vi "Main FPGA 5-axis Servo 2.vi"() -> ()   [LabVIEW 2014]
uses:
  <vilib>/Motion/MotorControl/_s/nism.interpretControlRegister.stateTransition.ctl
  <vilib>/Motion/MotorControl/_s/nism.encoder.config.ctl
  <vilib>/Motion/MotorControl/_s/nism.encoder.incremental.config.ctl
  <vilib>/Motion/MotorControl/_s/nism.incremental.indexCriteria.ctl
  <vilib>/Motion/MotorControl/_s/nism.mdoMemoryOffsets.ctl
  <vilib>/Motion/MotorControl/_s/nism.pid.gains.fxp.18.ctl
  <vilib>/Motion/MotorControl/_s/nism.pi.v.outputRange.fxp.6.12.ctl
  <vilib>/Platform/TimedLoop/XDataNode/timing_clust.ctl
  <vilib>/Platform/TimedLoop/XDataNode/nitl_modes.ctl
  <vilib>/Platform/TimedLoop/XDataNode/wakeup.ctl
  <vilib>/Motion/MotorControl/_s/nism.digitalInputs.portA.ctl
  <vilib>/rvi/Emulation/niFpgaGetClockAttributes.vi
  <vilib>/rvi/Emulation/niFpgaSctlEmulationGetInTimedLoop.vi
  <vilib>/rvi/Emulation/niFpgaEmulationReportErrorSimple.vi
  Global FPGA.vi
  <vilib>/Motion/MotorControl/_s/nism.interpretControlRegister.indexed.vi
  <vilib>/rvi/Emulation/niFpgaProcessEmulError.vi
  <vilib>/Motion/MotorControl/_s/nism.mdo.read.encoder.vi
  <vilib>/Motion/MotorControl/_s/nism.mdo.read.positionLoopSyncData.vi
  <vilib>/Motion/MotorControl/_s/nism.mdo.read.splineData.vi
  <vilib>/Motion/MotorControl/_s/nism.mdo.read.single.vi
  <vilib>/Motion/MotorControl/_s/nism.generateStatusRegister.indexed.vi
  <vilib>/rvi/eio/common/nirviEmuTemplateMethod_errors.vi
  <vilib>/rvi/Emulation/niFpgaCriticalErrorInLSC.vi
  <vilib>/Motion/MotorControl/_s/nism.splineInterpolation.fxp.3.vi
  <vilib>/Motion/MotorControl/_s/nism.pid.simple.fxp.2.vi
  <vilib>/Motion/MotorControl/_s/nism.mdo.handler.indexed.vi
  <vilib>/Motion/MotorControl/_s/nism.digitalFilter.indexed.vi
  <vilib>/Motion/MotorControl/_s/nism.interpretDIOControl.portA.multiple.vi
  <vilib>/Motion/MotorControl/_s/nism.generateDIOStatus.portA.indexed.2.vi
  <vilib>/Motion/SoftMotion/Synchronization/nism.rioScan.generateSyncScan.vi
  <vilib>/Motion/MotorControl/_s/nism.incremental.p.2.vi
  <vilib>/eio/EIONode/EIONode.xnode
  <vilib>/rvi/Analysis/measure/butterworth/XNode/niFpgaButterworthFilter.xnode
  <vilib>/Platform/TimedLoop/XDataNode/XDataNode.xnode
  <vilib>/Motion/MotorControl/NI_SoftMotion_MotorControlIP.lvlib
  <vilib>/Platform/TimedLoop/XDataNode/XDNodeRunTimeDep.lvlib
  <vilib>/Motion/SoftMotion/Synchronization/NI_SoftMotion_Synchronization.lvlib
panel:
  in  "Reset Encoder":bool caption="reset"
  out "corrected period":u16
  out "AO Check":fxp<+/-,20,5>
  in  "AO Disabled":bool
  out "x-y":u32
  out "pos. error exceeded":bool
  out "position error":i16
  in  "AO 3":fxp<+/-,20,5>
  in  "AO 2":fxp<+/-,20,5>
  in  "AO 1":fxp<+/-,20,5>
  in  "AO 0":fxp<+/-,20,5>
  in  "AO Override?":bool
  in  "output range":T1={"output low"=-8.0, "output high"=8.0}
  in  "gains":T2
  in  "position error limit":i16=10000
  out "SE value":u32 caption="value"
  in  "Memory Type":T3=90 caption="mbox memory offsets" items=["1 / Current Loop Rate"=108, "Anti-Resonance Enable Velocity"=98, "Axis Control Mode"=88, "Axis Velocity Filter Coefficient 1"=60, "Axis Velocity Filter Coefficient 2"=61, "Axis Velocity Filter Coefficient 3"=62, "Axis Velocity Filter Frequency"=59, "Captured Index Position"=68, "Captured Position"=58, "Coefficient 0"=96, "Coefficient 1"=95, "Coefficient 2"=101, "Coefficient 3"=97, "Coefficient 4"=99, "Coefficient 5"=100, "Compare Mode"=81, "Compare Period"=32, "Compare Position"=55, "Config Sent"=82, "Control Register"=33, "Control Register State Transition"=57, "Current Loop I2T Constant"=38, "Current Loop I2T Current to Clamp to"=40, "Current Loop I2T Icont Limit Squared"=39, "Current Loop Integral Gain"=36, "Current Loop Proportional Gain"=35, "Current Loop Rate"=37, "Digital Input Digital Filter"=1, "Digital Output Safe State"=73, "Encoder Filter Rate (uS)"=92, "Encoder Index Active State"=65, "Encoder Index Reference Line A State"=66, "Encoder Index Reference Line B State"=67, "Encoder Line A Active State"=63, "Encoder Line B Active State"=64, "Encoder Velocity"=90, "Enforce Open-Loop Position Error Limit"=71, "Fault Codes"=45, "Fault Occurred"=41, "Forward Limit Digital Filter"=24, "Gain Set 2 Current Loop Integral Gain"=106, "Gain Set 2 Current Loop Proportional Gain"=107, "Home Switch Digital Filter"=26, "Maximum Position Error Exceeded"=69, "Motor Hall Angle 1"=12, "Motor Hall Angle 2"=13, "Motor Hall Angle 3"=14, "Motor Peak Current"=16, "Motor Peak Time"=17, "Motor Phase Current Offset(A)"=83, "Motor Phase Current Offset(B)"=84, "Motor Poles"=18, "Motor Rated Phase Current"=15, "Null"=0, "PWM Periods Per Tick"=94, "Position Capture Active State"=56, "Position Capture Condition"=30, "Position Capture Digital Filter"=31, "Position Compare Action"=27, "Position Compare Active State"=54, "Position Compare Pulse Width"=29, "Position Compare Safe State"=72, "Position Compare Window"=28, "Position Loop Period"=103, "Position Loop Position Error Limit"=70, "Position Loop Proportional Gain"=9, "Reverse Limit Digital Filter"=25, "Scan Period (nsec)"=104, "Spline Period/Trajectory Period"=44, "Spline Type"=42, "Status Register"=34, "Stepper Current Reduction Delay"=20, "Stepper Current Reduction Percentage"=19, "Stepper Microstepping Rate"=21, "Stepper Minimum Pulse Width"=22, "Stepper Reduced Current"=85, "Stepper Spline Loop Period"=23, "Torque Smoothing Gain"=102, "Torque Smoothing Phase"=105, "Trajectory Period/Spline Period"=43]
  in  "Encoder filter value (us) Manual":u16=2000
  out "encoder config":T4
  in  "Velocity Filter Active?":bool
  in  "Encoder Config (Manual)":T4={"active states"={"line a active high?"=FALSE, "line b active high?"=FALSE, "index active high?"=FALSE}, "index criteria"={"a"=FALSE, "b"=FALSE, "z"=FALSE}, "vel. filter coeffs."=[0, 0, 0]} caption="encoder config"
  out "Home Limits":bool[](array[boolean])
  out "Fwd Limits":bool[](array[boolean])
  out "Rev Limits":bool[](array[boolean])
  out "Drive Enable":bool[](array[boolean])
  in  "Enable Watchdog":bool
  in  "Pet Watchdog":bool
  in  "Watchdog Timeout Period (ticks)":u64=40000000 format="%.0p"
  out "Watchdog Timed Out?":bool
  out "Time Since Last Pet":u64
  in  "Enable value":bool
  in  "Drive Enable override?":bool
  out "State":T7=enum."Start --> Initializing" caption="state transition"
  in  "Sync Value":bool
  in  "Sync Enable override?":bool
  in  "Invert direction?":bool
  out "Sync is Fault":bool
  out "Sync is Locked":bool
  # "Synchronization Loop"
  # "Control Status Loop"
  # "Notes: \n1. This VI provides the communication interface between the NI SoftMotion Engine and the LabVIEW FPGA Module. You must compile this VI for a specific FPGA target before use. After compiling, run the VI before running any of the Express VI examples. For information on moving this example to another FPGA target, refer to ni.com/info and enter info code fpgaex.\n\n2. Only use the Reset Axis button if you are unable to communicate with the axis by any other means. This button resets the device state machine and other VIs to a known state. After resetting the axis, switch the NI Scan Engine from Active Mode to Configuration Mode, then back to Active Mode, before attempting to enable the axis."
  # "(These two buttons \nare for testing\npurposes.)"
  # "(These two buttons \nare for testing\npurposes.)"
  # "Step/Direction Loop"
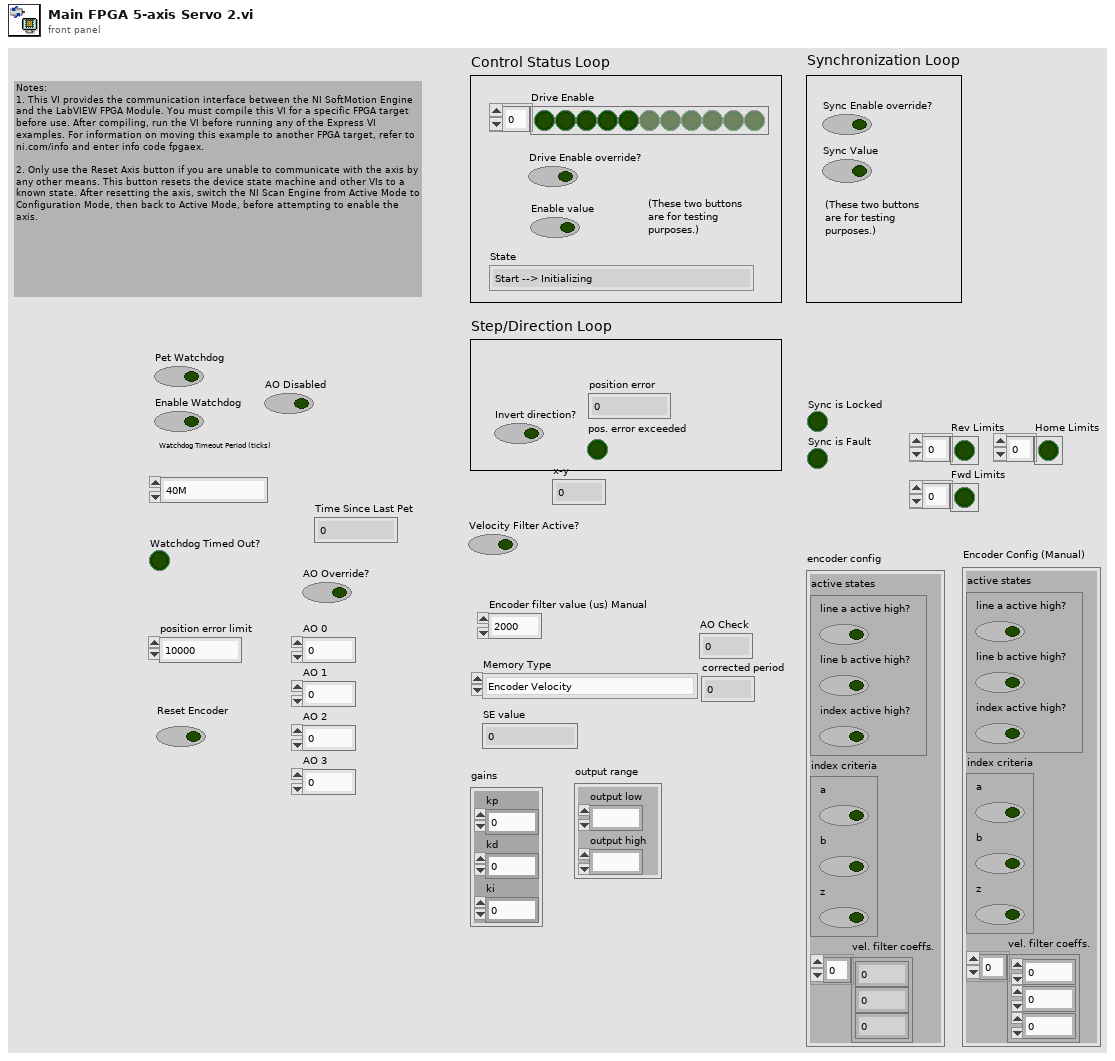
[diagram p1: front panel]
types:
  T1 = typedef "NI_SoftMotion_MotorControlIP.lvlib/nism.pi.v.outputRange.fxp.6.12.ctl" = cluster{"output low":fxp<+/-,18,6>, "output high":fxp<+/-,18,6>}
  T2 = typedef "NI_SoftMotion_MotorControlIP.lvlib/nism.pid.gains.fxp.18.ctl" = cluster{"kp":fxp<+,18,7>, "kd":fxp<+,18,7>, "ki":fxp<+,18,0>}
  T3 = typedef "NI_SoftMotion_MotorControlIP.lvlib/nism.mdoMemoryOffsets.ctl" = u16
  T4 = typedef "NI_SoftMotion_MotorControlIP.lvlib/nism.encoder.config.ctl" = cluster{"active states":T5, "index criteria":T6, "vel. filter coeffs.":i32[]}
  T5 = typedef "NI_SoftMotion_MotorControlIP.lvlib/nism.encoder.incremental.config.ctl" = cluster{"line a active high?":bool, "line b active high?":bool, "index active high?":bool}
  T6 = typedef "NI_SoftMotion_MotorControlIP.lvlib/nism.incremental.indexCriteria.ctl" = cluster{"a":bool, "b":bool, "z":bool}
  T7 = typedef "NI_SoftMotion_MotorControlIP.lvlib/nism.interpretControlRegister.stateTransition.ctl" = enum8{"Invalid", "Start --> Initializing", "Initializing --> Disabled", "Disabled --> Ready To Switch On", "Ready To Switch On --> Switched On", "Ready To Switch On --> Disable", "Switched On --> Operation Enable", "Switched On --> Ready To Switch On", "Switched On --> Disabled", "Operation Enable --> Switched On", "Operation Enable --> Ready To Switch On", "Operation Enable --> Disabled", "Fault --> Disabled", "Any --> Fault", "None"}
  T8 = typedef "NI_SoftMotion_Synchronization.lvlib/nism.softmotionScan.timerConfig.ctl" = cluster{"target period (clocks)":u16, "host period / target period":u16}
  T9 = typedef "NI_SoftMotion_Synchronization.lvlib/nism.softmotionScan.timerControl.ctl" = cluster{"sm scan":bool, "sm scan count":u32, "sm scan enabled":bool}
  T10 = typedef "NI_SoftMotion_MotorControlIP.lvlib/nism.mdo.splineData.ctl" = cluster{"spline type":T11, "traj per/spline per":u16, "spline per/traj per":fxp<+,32,0>}
  T11 = typedef "NI_SoftMotion_MotorControlIP.lvlib/nism.splineInterpolation.type.ctl" = u16
  T12 = typedef "NI_SoftMotion_MotorControlIP.lvlib/nism.digitalInputs.portA.ctl" = cluster{"reverse limit":bool, "forward limit":bool, "home switch":bool, "digital input 0":bool, "digital input 1":bool, "digital input 2":bool, "digital input 3":bool}
  T13 = typedef "NI_SoftMotion_MotorControlIP.lvlib/nism.dio.portA.config.2.ctl" = cluster{"digital filter (us)":u16[], "safe state":T14[]}
  T14 = typedef "nism.safeStates.ctl" = enum8{"Low", "High", "No Change"}
  T15 = typedef "XDNodeRunTimeDep.lvlib/timing_clust.ctl" = cluster{"Expected End [f-1]":u64, "Actual End [f-1]":u64, "Finished Late? [f-1]":bool, "Expected End [i-1]":u64, "Actual End [i-1]":u64, "Finished Late? [i-1]":bool, "Expected Start [i]":u64, "Actual Start [i]":u64, "Expected Start [f]":u64, "Actual Start [f]":u64, "Source Name":string, "Structure Name":string, "Period":i64, "Deadline":i64, "Offset":i64, "Start":i64, "Priority":i32, "Timeout":i32, "Mode":T16, "Wakeup Reason":T17, "Error":errorcluster, "Source Type":string, "Secondary Source Type":string, "Global End Time":u64, "Global Start Time":u64, "Frame Duration":u64, "Iteration Duration":u64, "Assigned CPU":i32, "I/O Scan Engine Mode":u32}
  T16 = typedef "XDNodeRunTimeDep.lvlib/nitl_modes.ctl" = enum32{"No Change", "Process missed periods, maintain original phase", "Discard missed periods, maintain original phase", "Process missed periods, ignore original phase", "Discard missed periods, ignore original phase"}
  T17 = typedef "XDNodeRunTimeDep.lvlib/wakeup.ctl" = enum32{"Normal", "Aborted", "Asynchronous wakeup", "Timing source error", "Timed loop error", "Timeout"}
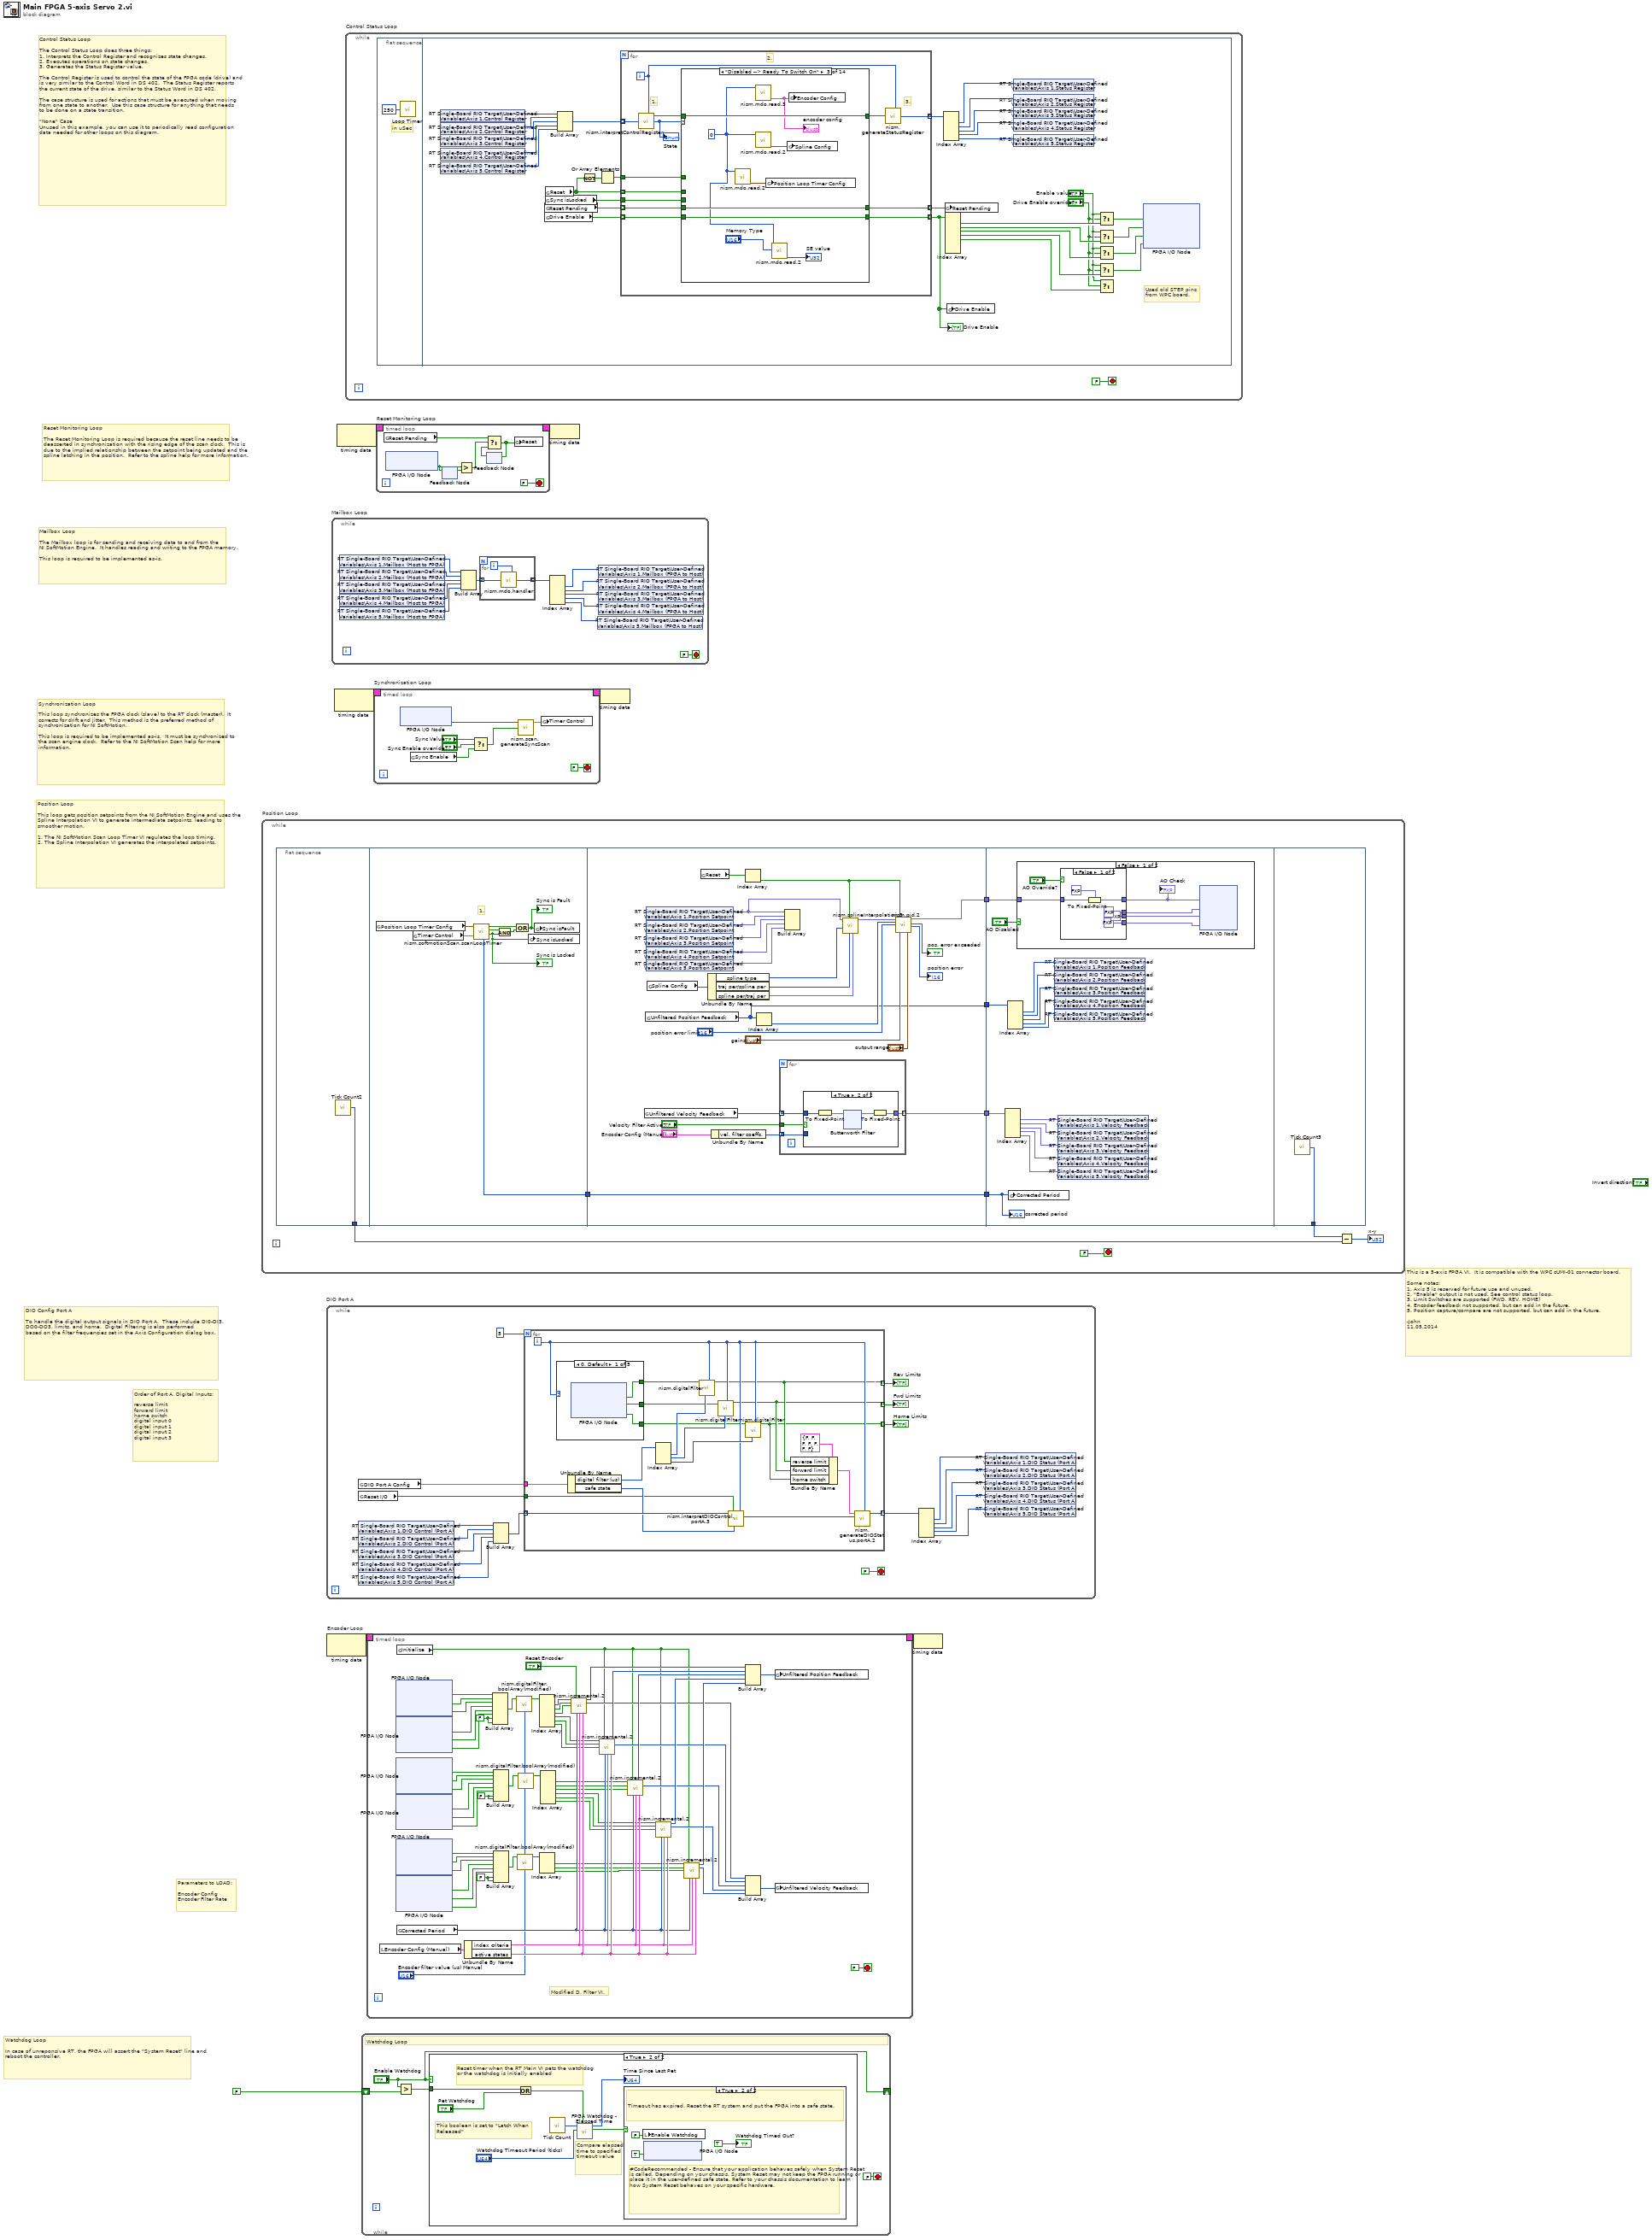
[diagram p0: block diagram]
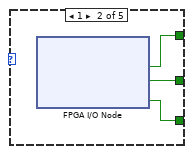
[diagram p2: hidden frame]
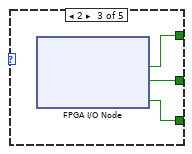
[diagram p3: hidden frame]
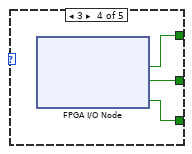
[diagram p4: hidden frame]
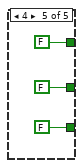
[diagram p5: hidden frame]
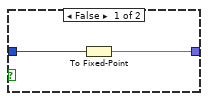
[diagram p8: hidden frame]
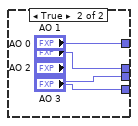
[diagram p9: hidden frame]
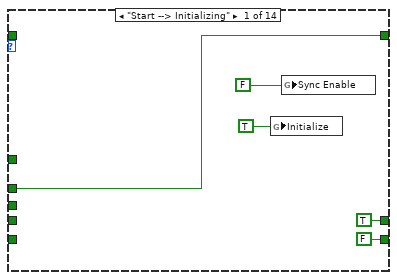
[diagram p11: hidden frame]
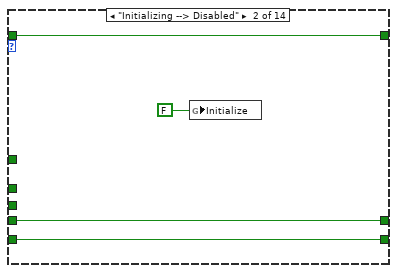
[diagram p12: hidden frame]
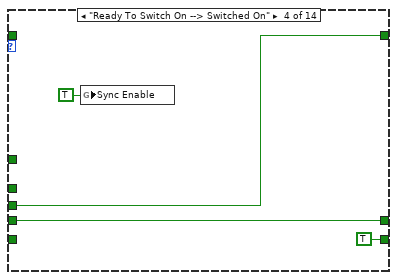
[diagram p13: hidden frame]
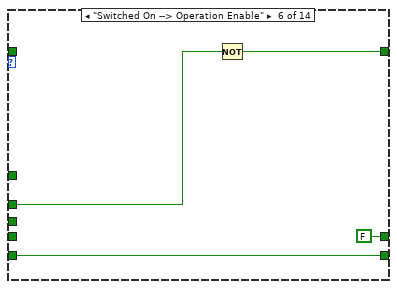
[diagram p15: hidden frame]
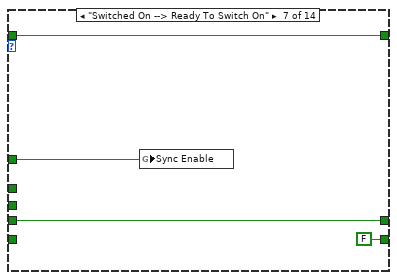
[diagram p16: hidden frame]
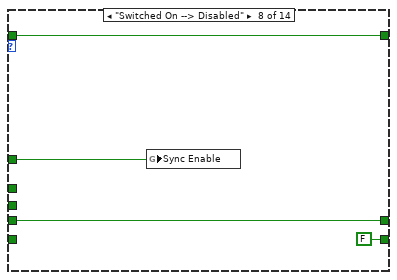
[diagram p17: hidden frame]
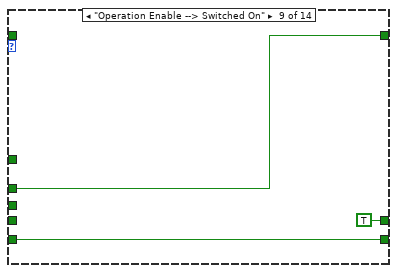
[diagram p18: hidden frame]
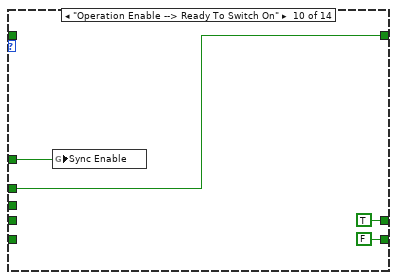
[diagram p19: hidden frame]
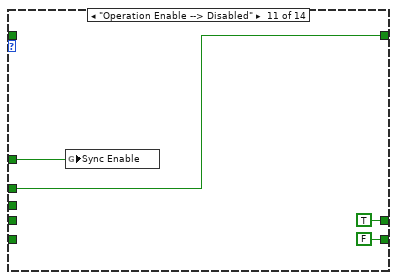
[diagram p20: hidden frame]
diagram:
  # "Parameters to LOAD:\n\nEncoder Config\nEncoder Filter Rate"
  # "This is a 5-axis FPGA VI.  It is compatible with the WPC cUMI-01 connector board.\n\nSome notes:\n1. Axis 5 is reserved for future use and unused.\n2. \"Enable\" output is not used. See control status loop.\n3. Limit Switches are supported (FWD, REV, HOME)\n4. Encoder feedback not supported, but can add in the future.\n5. Position capture/compare are not supported, but can add in the future.\n\n-John\n11.05.2014"
  # "DIO Config Port A\n\nTo handle the digital output signals in DIO Port A.  These include DI0-DI3, DO0-DO3, limits, and home.  Digital Filtering is also performed\nbased on the filter frequencies set in the Axis Configuration dialog box."
  # "Order of Port A, Digital Inputs:\n\nreverse limit\nforward limit\nhome switch\ndigital input 0\ndigital input 1\ndigital input 2\ndigital input 3"
  # "Watchdog Loop\n\nIn case of unreponsive RT, the FPGA will assert the \"System Reset\" line and reboot the controller."
  # "Position Loop\n\nThis loop gets position setpoints from the NI SoftMotion Engine and uses the Spline Interpolation VI to generate intermediate setpoints, leading to smoother motion.\n\n1. The NI SoftMotion Scan Loop Timer VI regulates the loop timing. \n2. The Spline Interpolation VI generates the interpolated setpoints."
  # "Synchronization Loop\n\nThis loop synchronizes the FPGA clock (slave) to the RT clock (master).  It corrects for drift and jitter.  This method is the preferred method of synchronization for NI SoftMotion.\n\nThis loop is required to be implemented as-is.  It must be synchronized to the scan engine clock.  Refer to the NI SoftMotion Scan help for more information."
  # "Mailbox Loop\n\nThe Mailbox loop is for sending and receiving data to and from the \nNI SoftMotion Engine.  It handles reading and writing to the FPGA memory.\n\nThis loop is required to be implemented as-is."
  # "Reset Monitoring Loop\n\nThe Reset Monitoring Loop is required because the reset line needs to be deasserted in synchronization with the rising edge of the scan clock.  This is due to the implied relationship between the setpoint being updated and the spline latching in the position.  Refer to the spline help for more information."
  # "Control Status Loop\n\nThe Control Status Loop does three things:\n1. Interprets the Control Register and recognizes state changes.\n2. Executes operations on state changes.\n3. Generates the Status Register value.\n\nThe Control Register is used to control the state of the FPGA code (drive) and is very similar to the Control Word in DS 402.  The Status Register reports the current state of the drive, similar to the Status Word in DS 402.\n\nThe case structure is used for actions that must be executed when moving from one state to another.  Use this case structure for anything that needs to be done on a state transition.\n\n\"None\" Case\nUnused in this example, you can use it to periodically read configuration data needed for other loops on this diagram."
  n1 = while "Position Loop" {
    stop <- FALSE stop-if-true
    n2 = flat-sequence {
      tunnel: [w17] -> w10
      tunnel: [w18] -> w14
      tunnel: [w46] -> w15
      tunnel: w14 -> [w46]
      tunnel: [w27] -> w13
      tunnel: [w39] -> w12
      tunnel: [w26] -> w8
      tunnel: w15 -> [w85]
      tunnel: w13 -> [w84]
      tunnel: w12 -> [w78]
      tunnel: w8 -> [w72]
      tunnel: [w102] -> w11
      frame #0 {
        n3 = call "Tick Count2"() -> ("Tick Count(Ticks)"=w17:u32)
      }
      frame #1 {
        # "1."
        n4 = global read "Global FPGA.vi" "Position Loop Timer Config"() -> (w20:T8)
        n5 = global read "Global FPGA.vi" "Timer Control"() -> (w19:T9)
        n6 = call <vilib>:"nism.softmotionScan.scanLoopTimer.vi"("timer control"=w19, "timer config"=w20) -> ("scan running?"=w22:bool, "finished late?"=w24:bool, "fault occurred?"=w25:bool, "corrected period"=w18:u16)  [unwired: 5 in, 1 out]
        "Sync is Locked" <- w22
        n7 = Compound Arithmetic op=AND(w24, w22) -> (w23:bool)
        n8 = Compound Arithmetic op=OR(w25, w23) -> (w21:bool)
        "Sync is Fault" <- w21
        n9 = global write "Global FPGA.vi" "Sync isLocked"(w22) -> ()
        n10 = global write "Global FPGA.vi" "Sync isFault"(w21) -> ()
      }
      frame #2 {
        n11 = global read "Global FPGA.vi" "Unfiltered Velocity Feedback"() -> (w40:i16[])
        n12 = global read "Global FPGA.vi" "Unfiltered Position Feedback"() -> (w27:i32[])
        n13 = shared-variable "RT Single-Board RIO Target\\User-Defined Variables\\Axis 1.Position Setpoint"() -> (w30:fxp<+/-,64,32>)  [unwired: 1 in, 1 out]
        n14 = shared-variable "RT Single-Board RIO Target\\User-Defined Variables\\Axis 2.Position Setpoint"() -> (w45:fxp<+/-,64,32>)  [unwired: 1 in, 1 out]
        n15 = shared-variable "RT Single-Board RIO Target\\User-Defined Variables\\Axis 3.Position Setpoint"() -> (w44:fxp<+/-,64,32>)  [unwired: 1 in, 1 out]
        n16 = shared-variable "RT Single-Board RIO Target\\User-Defined Variables\\Axis 4.Position Setpoint"() -> (w43:fxp<+/-,64,32>)  [unwired: 1 in, 1 out]
        n17 = shared-variable "RT Single-Board RIO Target\\User-Defined Variables\\Axis 5.Position Setpoint"() -> (w42:fxp<+/-,64,32>)  [unwired: 1 in, 1 out]
        n18 = global read "Global FPGA.vi" "Spline Config"() -> (w48:T10)
        n19 = global read "Global FPGA.vi" "Reset"() -> (w32:bool[])
        n20 = Unbundle By Name(w48) -> ("spline type"=w51:T11, "traj per/spline per"=w50:u16, "spline per/traj per"=w49:fxp<+,32,0>)
        n21 = Unbundle By Name("Encoder Config (Manual)") -> ("vel. filter coeffs."=w41:i32[])
        n22 = Index Array(array=w32) -> (element=w31:bool)  [unwired: 1 in]
        n23 = Index Array(array=w27) -> (element=w33:i32)  [unwired: 1 in]
        n24 = for {
          tunnel: "Velocity Filter Active?" -> [w55]
          tunnel: w41 -> [w54] mode=indexing
          tunnel: w40 -> [w53] mode=indexing
          tunnel: [w52] -> w39 mode=indexing
          n25 = case shown="True" w55 {
            tunnel: w53 -> [w57 w61]
            tunnel: w54 -> [_ _]
            tunnel: [w56 w59] -> w52
            frame False {
              n26 = To Fixed-Point(number=w57) -> (fixed-point=w56:fxp<+/-,64,32>)  [unwired: 1 in]
            }
            frame True {
              n27 = To Fixed-Point(number=w61) -> (fixed-point=w60:fxp<+/-,16,16>)  [unwired: 1 in]
              n28 = xnode "Butterworth Filter"("input data"=w60) -> ("output data"=w58:fxp<+/-,16,16>)  [unwired: 2 in, 1 out]
              n29 = To Fixed-Point(number=w58) -> (fixed-point=w59:fxp<+/-,64,32>)  [unwired: 1 in]
            }
          }
        }
        n30 = Build Array(w30, w45, w44, w43, w42) -> ()  [unwired: 1 out]
        n31 = call-poly <vilib>:"nism.splineInterpolation.3.vi"("1 / calls per sample"=w49, "calls per sample"=w50, "reset"=w31, "spline type"=w51, "x"=w30) -> ("xi"=w47:fxp<+/-,64,32>)  [unwired: 5 in, 1 out]
        n32 = call-poly <vilib>:"nism.pid.2.vi"("position setpoint"=w47, "position feedback"=w33, "position error limit"="position error limit", "reset"=w31, "gains"="gains", "output range"="output range") -> ("current setpoint"=w26:fxp<+/-,18,6>, "pos. error exceeded"=→"pos. error exceeded":bool, "position error"=→"position error":i16)  [unwired: 11 in]
      }
      frame #3 {
        n33 = Index Array(array=w78) -> (element #1=w77:fxp<+/-,64,32>, element #2=w76:fxp<+/-,64,32>, element #3=w75:fxp<+/-,64,32>, element #4=w74:fxp<+/-,64,32>, element #5=w73:fxp<+/-,64,32>)  [unwired: 5 in]
        n34 = Index Array(array=w84) -> (element #1=w83:i32, element #2=w82:i32, element #3=w81:i32, element #4=w80:i32, element #5=w79:i32)  [unwired: 5 in]
        n35 = global write "Global FPGA.vi" "Corrected Period"(w85) -> ()
        n36 = case shown="False" "AO Disabled" {
          tunnel: w72 -> [w86 _]
          frame False {
            n37 = case shown="False" "AO Override?" {
              tunnel: [w93 "AO 0"] -> w90
              tunnel: [fxp<+/-,20,5> 0.0 ("AO 1") "AO 1"] -> w89
              tunnel: [fxp<+/-,20,5> 0.0 ("AO 2") "AO 2"] -> w88
              tunnel: [fxp<+/-,20,5> 0.0 ("AO 3") "AO 3"] -> w87
              tunnel: w86 -> [w92 _]
              frame False {
                n38 = To Fixed-Point(fixed-point type=fxp<+/-,20,5> 0.0 ("AO 1"), number=w92) -> (fixed-point=w93:fxp<+/-,20,5>)
              }
              frame True {
              }
            }
            "AO Check" <- w90
            n39 = xnode "FPGA I/O Node"("AO0"=w90, "AO1"=w89, "AO2"=w88, "AO3"=w87) -> ()  [unwired: 4 in, 4 out]
          }
          frame True {
          }
        }
        n40 = shared-variable "RT Single-Board RIO Target\\User-Defined Variables\\Axis 1.Position Feedback"(w83) -> ()  [unwired: 1 in, 1 out]
        n41 = shared-variable "RT Single-Board RIO Target\\User-Defined Variables\\Axis 2.Position Feedback"(w82) -> ()  [unwired: 1 in, 1 out]
        n42 = shared-variable "RT Single-Board RIO Target\\User-Defined Variables\\Axis 3.Position Feedback"(w81) -> ()  [unwired: 1 in, 1 out]
        n43 = shared-variable "RT Single-Board RIO Target\\User-Defined Variables\\Axis 4.Position Feedback"(w80) -> ()  [unwired: 1 in, 1 out]
        n44 = shared-variable "RT Single-Board RIO Target\\User-Defined Variables\\Axis 5.Position Feedback"(w79) -> ()  [unwired: 1 in, 1 out]
        n45 = shared-variable "RT Single-Board RIO Target\\User-Defined Variables\\Axis 1.Velocity Feedback"(w77) -> ()  [unwired: 1 in, 1 out]
        n46 = shared-variable "RT Single-Board RIO Target\\User-Defined Variables\\Axis 2.Velocity Feedback"(w76) -> ()  [unwired: 1 in, 1 out]
        n47 = shared-variable "RT Single-Board RIO Target\\User-Defined Variables\\Axis 3.Velocity Feedback"(w75) -> ()  [unwired: 1 in, 1 out]
        n48 = shared-variable "RT Single-Board RIO Target\\User-Defined Variables\\Axis 4.Velocity Feedback"(w74) -> ()  [unwired: 1 in, 1 out]
        n49 = shared-variable "RT Single-Board RIO Target\\User-Defined Variables\\Axis 5.Velocity Feedback"(w73) -> ()  [unwired: 1 in, 1 out]
        "corrected period" <- w85
      }
      frame #4 {
        n50 = call "Tick Count3"() -> ("Tick Count(Ticks)"=w102:u32)
      }
    }
    n51 = Subtract(x=w11, y=w10) -> (x-y=→"x-y":u32)
  }
  n52 = while "DIO Port A" {
    stop <- FALSE stop-if-true
    n53 = global read "Global FPGA.vi" "DIO Port A Config"() -> (w120:T13)
    n54 = global read "Global FPGA.vi" "Reset I/O"() -> (w119:bool)
    n55 = shared-variable "RT Single-Board RIO Target\\User-Defined Variables\\Axis 1.DIO Control (Port A)"() -> (w117:u32)  [unwired: 1 in, 1 out]
    n56 = shared-variable "RT Single-Board RIO Target\\User-Defined Variables\\Axis 2.DIO Control (Port A)"() -> (w116:u32)  [unwired: 1 in, 1 out]
    n57 = shared-variable "RT Single-Board RIO Target\\User-Defined Variables\\Axis 3.DIO Control (Port A)"() -> (w115:u32)  [unwired: 1 in, 1 out]
    n58 = shared-variable "RT Single-Board RIO Target\\User-Defined Variables\\Axis 4.DIO Control (Port A)"() -> (w114:u32)  [unwired: 1 in, 1 out]
    n59 = shared-variable "RT Single-Board RIO Target\\User-Defined Variables\\Axis 5.DIO Control (Port A)"() -> (w113:u32)  [unwired: 1 in, 1 out]
    n60 = Build Array(w117, w116, w115, w114, w113) -> (w112:u32[])
    n61 = for {
      N: 5 -> [_]
      tunnel: [w139] -> w106 mode=indexing
      tunnel: w112 -> [w138] mode=indexing
      tunnel: w120 -> [w135]
      tunnel: w119 -> [w133]
      tunnel: [w124] -> w105 mode=indexing
      tunnel: [w123] -> w104 mode=indexing
      tunnel: [w122] -> w103 mode=indexing
      i -> [w128]
      n62 = case shown="0, Default" w128 {
        tunnel: [w143 w146 w149 w152 FALSE ("RMC/DIO44")] -> w127
        tunnel: [w141 w144 w147 w150 FALSE ("RMC/DIO61")] -> w126
        tunnel: [w142 w145 w148 w151 FALSE ("RMC/DIO77")] -> w125
        frame 0, Default {
          n63 = xnode "FPGA I/O Node"() -> ("RMC/DIO29"=w143:bool, "RMC/DIO93"=w142:bool, "RMC/DIO11"=w141:bool)  [unwired: 3 in, 3 out]
        }
        frame 1 {
          n64 = xnode "FPGA I/O Node"() -> ("RMC/DIO44"=w146:bool, "RMC/DIO77"=w145:bool, "RMC/DIO61"=w144:bool)  [unwired: 3 in, 3 out]
        }
        frame 2 {
          n65 = xnode "FPGA I/O Node"() -> ("RMC/DIO31"=w149:bool, "RMC/DIO95"=w148:bool, "RMC/DIO13"=w147:bool)  [unwired: 3 in, 3 out]
        }
        frame 3 {
          n66 = xnode "FPGA I/O Node"() -> ("RMC/DIO47"=w152:bool, "RMC/DIO46"=w151:bool, "RMC/DIO79"=w150:bool)  [unwired: 3 in, 3 out]
        }
        frame 4 {
        }
      }
      n67 = Unbundle By Name(w135) -> ("digital filter (us)"=w129:u16[], "safe state"=w134:T14[])
      n68 = Index Array(array=w129) -> (element #1=w130:u16, element #2=w131:u16, element #3=w132:u16)  [unwired: 3 in]
      n69 = call-poly <vilib>:"nism.digitalFilter.vi"("index"=w128, "filter value (us)"=w130, "input signal"=w127) -> ("output signal"=w124:bool)  [unwired: 8 in]
      n70 = call-poly <vilib>:"nism.digitalFilter.vi"("index"=w128, "filter value (us)"=w131, "input signal"=w125) -> ("output signal"=w123:bool)  [unwired: 8 in]
      n71 = call-poly <vilib>:"nism.interpretDIOControl.portA.3.vi"("index"=w128, "safe state"=w134, "reset"=w133, "dio control(port a)"=w138) -> ("reset latches"=w140:u8)  [unwired: 6 in, 1 out]
      n72 = call-poly <vilib>:"nism.digitalFilter.vi"("index"=w128, "filter value (us)"=w132, "input signal"=w126) -> ("output signal"=w122:bool)  [unwired: 8 in]
      n73 = Bundle By Name(cluster=T12 {"reverse limit"=FALSE, "forward limit"=FALSE, "home switch"=FALSE, "digital input 0"=FALSE, "digital input 1"=FALSE, "digital input 2"=FALSE, "digital input 3"=FALSE} ("$(driveInterface.digitalInputs.shortName)"), "reverse limit"=w124, "forward limit"=w123, "home switch"=w122) -> (w136:T12)
      n74 = call-poly <vilib>:"nism.generateDIOStatus.portA.2.vi"("index"=w128, "reset latches"=w140, "digital inputs"=w136) -> ("dio status(port a)"=w139:u32)  [unwired: 8 in]
    }
    "Rev Limits" <- w105
    "Fwd Limits" <- w104
    "Home Limits" <- w103
    n75 = Index Array(array=w106) -> (element #1=w111:u32, element #2=w110:u32, element #3=w109:u32, element #4=w108:u32, element #5=w107:u32)  [unwired: 5 in]
    n76 = shared-variable "RT Single-Board RIO Target\\User-Defined Variables\\Axis 1.DIO Status (Port A)"(w111) -> ()  [unwired: 1 in, 1 out]
    n77 = shared-variable "RT Single-Board RIO Target\\User-Defined Variables\\Axis 2.DIO Status (Port A)"(w110) -> ()  [unwired: 1 in, 1 out]
    n78 = shared-variable "RT Single-Board RIO Target\\User-Defined Variables\\Axis 3.DIO Status (Port A)"(w109) -> ()  [unwired: 1 in, 1 out]
    n79 = shared-variable "RT Single-Board RIO Target\\User-Defined Variables\\Axis 4.DIO Status (Port A)"(w108) -> ()  [unwired: 1 in, 1 out]
    n80 = shared-variable "RT Single-Board RIO Target\\User-Defined Variables\\Axis 5.DIO Status (Port A)"(w107) -> ()  [unwired: 1 in, 1 out]
  }
  n81 = node-c288() -> (w2:T15)  [unwired: 1 in]
  n82 = while "Mailbox Loop" {
    stop <- FALSE stop-if-true
    n83 = shared-variable "RT Single-Board RIO Target\\User-Defined Variables\\Axis 1.Mailbox (Host to FPGA)"() -> (w165:u64)  [unwired: 1 in, 1 out]
    n84 = shared-variable "RT Single-Board RIO Target\\User-Defined Variables\\Axis 2.Mailbox (Host to FPGA)"() -> (w164:u64)  [unwired: 1 in, 1 out]
    n85 = shared-variable "RT Single-Board RIO Target\\User-Defined Variables\\Axis 3.Mailbox (Host to FPGA)"() -> (w163:u64)  [unwired: 1 in, 1 out]
    n86 = shared-variable "RT Single-Board RIO Target\\User-Defined Variables\\Axis 4.Mailbox (Host to FPGA)"() -> (w162:u64)  [unwired: 1 in, 1 out]
    n87 = shared-variable "RT Single-Board RIO Target\\User-Defined Variables\\Axis 5.Mailbox (Host to FPGA)"() -> (w161:u64)  [unwired: 1 in, 1 out]
    n88 = Build Array(w165, w164, w163, w162, w161) -> (w167:u64[])
    n89 = for {
      tunnel: w167 -> [w171] mode=indexing
      tunnel: [w170] -> w166 mode=indexing
      i -> [w169]
      n90 = call-poly <vilib>:"nism.mdo.handler.vi"("mbox (host to fpga)"=w171, "axis index"=w169) -> ("mbox (fpga to host)"=w170:u64)  [unwired: 7 in]
    }
    n91 = Index Array(array=w166) -> (element #1=w160:u64, element #2=w159:u64, element #3=w158:u64, element #4=w157:u64, element #5=w156:u64)  [unwired: 5 in]
    n92 = shared-variable "RT Single-Board RIO Target\\User-Defined Variables\\Axis 5.Mailbox (FPGA to Host)"(w156) -> ()  [unwired: 1 in, 1 out]
    n93 = shared-variable "RT Single-Board RIO Target\\User-Defined Variables\\Axis 1.Mailbox (FPGA to Host)"(w160) -> ()  [unwired: 1 in, 1 out]
    n94 = shared-variable "RT Single-Board RIO Target\\User-Defined Variables\\Axis 2.Mailbox (FPGA to Host)"(w159) -> ()  [unwired: 1 in, 1 out]
    n95 = shared-variable "RT Single-Board RIO Target\\User-Defined Variables\\Axis 3.Mailbox (FPGA to Host)"(w158) -> ()  [unwired: 1 in, 1 out]
    n96 = shared-variable "RT Single-Board RIO Target\\User-Defined Variables\\Axis 4.Mailbox (FPGA to Host)"(w157) -> ()  [unwired: 1 in, 1 out]
  }
  n97 = node-c288() -> (w7:T15)  [unwired: 1 in]
  n98 = node-c288() -> (w5:T15)  [unwired: 1 in]
  n99 = while "Control Status Loop" {
    stop <- FALSE stop-if-true
    n100 = flat-sequence {
      frame #0 {
        # "in uSec"
        n101 = call "Loop Timer"("Count(uSec)"=u32 250) -> ()  [unwired: 1 out]
      }
      frame #1 {
        # "Used old STEP pins\nfrom WPC board."
        n102 = shared-variable "RT Single-Board RIO Target\\User-Defined Variables\\Axis 1.Control Register"() -> (w194:u32)  [unwired: 1 in, 1 out]
        n103 = shared-variable "RT Single-Board RIO Target\\User-Defined Variables\\Axis 2.Control Register"() -> (w193:u32)  [unwired: 1 in, 1 out]
        n104 = shared-variable "RT Single-Board RIO Target\\User-Defined Variables\\Axis 3.Control Register"() -> (w192:u32)  [unwired: 1 in, 1 out]
        n105 = shared-variable "RT Single-Board RIO Target\\User-Defined Variables\\Axis 4.Control Register"() -> (w191:u32)  [unwired: 1 in, 1 out]
        n106 = shared-variable "RT Single-Board RIO Target\\User-Defined Variables\\Axis 5.Control Register"() -> (w190:u32)  [unwired: 1 in, 1 out]
        n107 = global read "Global FPGA.vi" "Reset Pending"() -> (w198:bool[])
        n108 = global read "Global FPGA.vi" "Drive Enable"() -> (w197:bool[])
        n109 = global read "Global FPGA.vi" "Reset"() -> (w199:bool[])
        n110 = global read "Global FPGA.vi" "Sync isLocked"() -> (w204:bool)
        n111 = Build Array(w194, w193, w192, w191, w190) -> (w203:u32[])
        n112 = Not(x=w199) -> (.not. x?=w201:bool[])
        n113 = Or Array Elements(Boolean array=w201) -> (logical OR=w200:bool)
        n114 = for {
          tunnel: w199 -> [w212] mode=indexing
          tunnel: w204 -> [w211]
          tunnel: w203 -> [w213] mode=indexing
          tunnel: [w210] -> w195 mode=indexing
          tunnel: [w209] -> w202 mode=indexing
          tunnel: [w208] -> w196 mode=indexing
          tunnel: w200 -> [w207]
          tunnel: w198 -> [w206] mode=indexing
          tunnel: w197 -> [w205] mode=indexing
          i -> [w214]
          # "3."
          # "2."
          # "1."
          n115 = call-poly <vilib>:"nism.interpretControlRegister.vi"("control register"=w213, "axis index"=w214) -> ("transition occurred"=w215:bool, "state transition"=w216:T7)  [unwired: 6 in]
          "State" <- w216
          n116 = case shown="\"Disabled --> Ready To Switch On\"" w216 {
            tunnel: w215 -> [_ w226 w235 _ w242 _ w250 w254 _ _ _ _ w274 _]
            tunnel: [w222 w226 w235 w237 w242 w246 w250 w254 w256 w259 w263 w267 w273 _] -> w217
            tunnel: w212 -> [w222 _ _ _ _ w245 _ _ w256 w259 w263 w267 _ _]
            tunnel: w211 -> [_ _ _ w237 _ _ _ _ _ _ _ _ _ _]
            tunnel: [TRUE ("Write.Reset Pending") w225 w232 w236 w241 FALSE ("Write.Reset Pending") w247 w251 TRUE ("Write.Reset Pending") TRUE ("Write.Reset Pending") TRUE ("Write.Reset Pending") TRUE ("Write.Reset Pending") w271 w276] -> w209
            tunnel: [FALSE ("Write.Drive Enable") w224 w231 TRUE ("Write.Drive Enable") w240 w243 FALSE ("Write.Drive Enable") FALSE ("Write.Drive Enable") w255 FALSE ("Write.Drive Enable") FALSE ("Write.Drive Enable") FALSE ("Write.Drive Enable") w270 w275] -> w208
            tunnel: w207 -> [_ _ _ _ _ _ w248 w252 _ w258 w262 w266 w272 _]
            tunnel: w206 -> [_ w225 w232 w236 w241 _ w247 w251 _ _ _ _ w271 w276]
            tunnel: w205 -> [_ w224 w231 _ w240 w243 _ _ w255 _ _ _ w270 w275]
            frame "Start --> Initializing" {
              n117 = global write "Global FPGA.vi" "Initialize"(TRUE ("Initialize")) -> ()
              n118 = global write "Global FPGA.vi" "Sync Enable"(FALSE ("Sync Enable")) -> ()
            }
            frame "Initializing --> Disabled" {
              n119 = global write "Global FPGA.vi" "Initialize"(FALSE ("Initialize")) -> ()
            }
            frame "Disabled --> Ready To Switch On" {
              w227 = 0 ("axis index")
              n120 = call-poly <vilib>:"nism.mdo.read.2.vi"("axis index"=w227) -> ("position loop sync"=w233:T8)  [unwired: 10 in]
              n121 = call-poly <vilib>:"nism.mdo.read.3.vi"("axis index"=w227) -> ("encoder config"=w230:T4)  [unwired: 10 in]
              "encoder config" <- w230
              n122 = call-poly <vilib>:"nism.mdo.read.2.vi"("axis index"=w227) -> ("spline"=w234:T10)  [unwired: 10 in]
              n123 = global write "Global FPGA.vi" "Position Loop Timer Config"(w233) -> ()
              n124 = call-poly <vilib>:"nism.mdo.read.2.vi"("mbox memory offsets"="Memory Type", "axis index"=w227) -> ("value"=→"SE value":u32)  [unwired: 9 in]
              n125 = global write "Global FPGA.vi" "Spline Config"(w234) -> ()
              n126 = global write "Global FPGA.vi" "Encoder Config"(w230) -> ()
            }
            frame "Ready To Switch On --> Switched On" {
              n127 = global write "Global FPGA.vi" "Sync Enable"(TRUE ("Sync Enable")) -> ()
            }
            frame "Ready To Switch On --> Disable" {
            }
            frame "Switched On --> Operation Enable" {
              n128 = Not(x=w245) -> (.not. x?=w246:bool)
            }
            frame "Switched On --> Ready To Switch On" {
              n129 = global write "Global FPGA.vi" "Sync Enable"(w248) -> ()
            }
            frame "Switched On --> Disabled" {
              n130 = global write "Global FPGA.vi" "Sync Enable"(w252) -> ()
            }
            frame "Operation Enable --> Switched On" {
            }
            frame "Operation Enable --> Ready To Switch On" {
              n131 = global write "Global FPGA.vi" "Sync Enable"(w258) -> ()
            }
            frame "Operation Enable --> Disabled" {
              n132 = global write "Global FPGA.vi" "Sync Enable"(w262) -> ()
            }
            frame "Any --> Fault" {
              n133 = global write "Global FPGA.vi" "Sync Enable"(w266) -> ()
            }
            frame "Fault --> Disabled" {
              # "wait one cycle for clear faults to have taken effect"
              n134 = global write "Global FPGA.vi" "Sync Enable"(w272) -> ()
              n135 = Not(x=w274) -> (.not. x?=w273:bool)
            }
            frame "None", Default {
            }
          }
          n136 = call-poly <vilib>:"nism.generateStatusRegister.vi"("transition success"=w217, "axis index"=w214) -> ("status register"=w210:u32)  [unwired: 7 in]
        }
        "Drive Enable" <- w196
        n137 = Index Array(array=w195) -> (element #1=w189:u32, element #2=w188:u32, element #3=w187:u32, element #4=w186:u32, element #5=w185:u32)  [unwired: 5 in]
        n138 = global write "Global FPGA.vi" "Reset Pending"(w202) -> ()
        n139 = Index Array(array=w196) -> (element #1=w184:bool, element #2=w183:bool, element #3=w182:bool, element #4=w181:bool, element #5=w180:bool)  [unwired: 8 in, 3 out]
        n140 = global write "Global FPGA.vi" "Drive Enable"(w196) -> ()
        n141 = shared-variable "RT Single-Board RIO Target\\User-Defined Variables\\Axis 1.Status Register"(w189) -> ()  [unwired: 1 in, 1 out]
        n142 = shared-variable "RT Single-Board RIO Target\\User-Defined Variables\\Axis 2.Status Register"(w188) -> ()  [unwired: 1 in, 1 out]
        n143 = shared-variable "RT Single-Board RIO Target\\User-Defined Variables\\Axis 3.Status Register"(w187) -> ()  [unwired: 1 in, 1 out]
        n144 = shared-variable "RT Single-Board RIO Target\\User-Defined Variables\\Axis 4.Status Register"(w186) -> ()  [unwired: 1 in, 1 out]
        n145 = shared-variable "RT Single-Board RIO Target\\User-Defined Variables\\Axis 5.Status Register"(w185) -> ()  [unwired: 1 in, 1 out]
        n146 = Select(t="Enable value", s="Drive Enable override?", f=w184) -> (s? t:f=w177:bool)
        n147 = Select(t="Enable value", s="Drive Enable override?", f=w183) -> (s? t:f=w176:bool)
        n148 = Select(t="Enable value", s="Drive Enable override?", f=w182) -> (s? t:f=w175:bool)
        n149 = Select(t="Enable value", s="Drive Enable override?", f=w181) -> (s? t:f=w174:bool)
        n150 = Select(t="Enable value", s="Drive Enable override?", f=w180) -> ()  [unwired: 1 out]
        n151 = xnode "FPGA I/O Node"("RMC/DIO28"=w177, "RMC/DIO12"=w176, "RMC/DIO30"=w175, "RMC/DIO14"=w174) -> ()  [unwired: 4 in, 4 out]
      }
    }
  }
  n152 = while "RT Watchdog Loop" {
    shift-right: ["Enable Watchdog"] -> _
    shift-left: FALSE ("Enable RT Watchdog") -> [w280]
    stop <- FALSE stop-if-true
    # "Watchdog Loop"
    n153 = Greater?(x="Enable Watchdog", y=w280) -> (0:w277:bool)
    n154 = case shown="True" "Enable Watchdog" {
      tunnel: w277 -> [_ w283]
      frame False {
        # "This loop has to be explicitly enabled from the RT Main VI.  This reduces the possiblity of an endless reboot cycle."
      }
      frame True {
        # "This boolean is set to \"Latch When Released\""
        # "Compare elapsed time to specified timeout value"
        # "Reset timer when the RT Main VI pets the watchdog or the watchdog is initially enabled"
        n155 = Or(x=w283, y="Pet Watchdog") -> (x .or. y?=w282:bool)
        n156 = call "Tick Count"() -> ("Tick Count(Ticks)"=w286:u32)
        n157 = call "FPGA Watchdog - Elapsed Time.vi"("Reset"=w282, "Timeout Period"="Watchdog Timeout Period (ticks)", "Current Time"=w286) -> ("Timeout"=w281:bool, "Elapsed Time"=→"Time Since Last Pet":u64)  [unwired: 7 in]
        n158 = case shown="True" w281 {
          frame False {
            # "Timeout has not expired."
          }
          frame True {
            # "#CodeRecommended - Ensure that your application behaves safely when System Reset is called. Depending on your chassis, System Reset may not keep the FPGA running or place it in the user-defined safe state. Refer to your chassis documentation to learn how System Reset behaves on your specific hardware."
            # "Timeout has expired. Reset the RT system and put the FPGA into a safe state."
            n159 = local write "Enable Watchdog"(FALSE ("Enable RT Watchdog")) -> ()
            n160 = xnode "FPGA I/O Node"("System Reset"=TRUE ("RT Reset on Watchdog Failure?")) -> ()  [unwired: 1 in, 1 out]
            "Watchdog Timed Out?" <- TRUE ("Watchdog Timed Out?")
          }
        }
      }
    }
  }
  n161 = timed-loop "Encoder Loop" {
    timing: w2 -> [_]
    timing-out: [_] -> w1
    stop <- FALSE stop-if-true
    w306 = FALSE ("element")
    w307 = FALSE ("element")
    w323 = FALSE ("element")
    # "Modified D. Filter VI."
    n162 = local read "Encoder Config (Manual)"() -> (w293:T4)
    n163 = xnode "FPGA I/O Node"() -> ("RMC/DIO60"=w350:bool, "RMC/DIO42"=w351:bool, "RMC/DIO75"=w349:bool)  [unwired: 3 in, 3 out]
    n164 = xnode "FPGA I/O Node"() -> ("RMC/DIO59"=w328:bool, "RMC/DIO92"=w327:bool, "RMC/DIO10"=w326:bool)  [unwired: 3 in, 3 out]
    n165 = xnode "FPGA I/O Node"() -> ("RMC/DIO74"=w319:bool, "RMC/DIO27"=w318:bool, "RMC/DIO91"=w317:bool)  [unwired: 3 in, 3 out]
    n166 = xnode "FPGA I/O Node"() -> ("RMC/DIO9"=w316:bool, "RMC/DIO41"=w315:bool, "RMC/DIO26"=w314:bool)  [unwired: 3 in, 3 out]
    n167 = xnode "FPGA I/O Node"() -> ("RMC/DIO58"=w300:bool, "RMC/DIO40"=w301:bool, "RMC/DIO73"=w302:bool)  [unwired: 3 in, 3 out]
    n168 = xnode "FPGA I/O Node"() -> ("RMC/DIO57"=w303:bool, "RMC/DIO90"=w304:bool, "RMC/DIO8"=w305:bool)  [unwired: 3 in, 3 out]
    n169 = global read "Global FPGA.vi" "Initialize"() -> (w294:bool)
    n170 = global read "Global FPGA.vi" "Corrected Period"() -> (w341:u16)
    n171 = Unbundle By Name(w293) -> ("index criteria"=w342:T6, "active states"=w343:T5)
    n172 = Build Array(w350, w351, w349, w328, w327, w326, w323, w323) -> (w348:bool[])
    n173 = Build Array(w300, w301, w302, w303, w304, w305, w306, w306) -> (w299:bool[])
    n174 = Build Array(w319, w318, w317, w316, w315, w314, w307, w307) -> (w324:bool[])
    n175 = call "nism.digitalFilter.boolArray(modified).vi"("filter value (us)"="Encoder filter value (us) Manual", "input signal"=w348) -> ("output signal"=w347:bool[])  [unwired: 9 in]
    n176 = call "nism.digitalFilter.boolArray(modified).vi"("filter value (us)"="Encoder filter value (us) Manual", "input signal"=w299) -> ("output signal"=w298:bool[])  [unwired: 9 in]
    n177 = call "nism.digitalFilter.boolArray(modified).vi"("filter value (us)"="Encoder filter value (us) Manual", "input signal"=w324) -> ("output signal"=w325:bool[])  [unwired: 9 in]
    n178 = Index Array(array=w347) -> (element #1=w346:bool, element #2=w345:bool, element #3=w344:bool, element #4=w322:bool, element #5=w321:bool, element #6=w320:bool)  [unwired: 6 in]
    n179 = Index Array(array=w298) -> (element #1=w297:bool, element #2=w296:bool, element #3=w295:bool)  [unwired: 3 in]
    n180 = Index Array(array=w325) -> (element #1=w313:bool, element #2=w312:bool, element #3=w311:bool, element #4=w310:bool, element #5=w309:bool, element #6=w308:bool)  [unwired: 6 in]
    n181 = call-poly <vilib>:"nism.incremental.2.vi"("a phase"=w346, "reset"="Reset Encoder", "b phase"=w345, "z phase"=w344, "calls per sample"=w341, "index criteria"=w342, "active states"=w343) -> ("encoder position"=w340:i32, "velocity"=w333:i16)  [unwired: 5 in, 2 out]
    n182 = call-poly <vilib>:"nism.incremental.2.vi"("a phase"=w322, "reset"=w294, "b phase"=w321, "z phase"=w320, "calls per sample"=w341, "index criteria"=w342, "active states"=w343) -> ("encoder position"=w339:i32, "velocity"=w332:i16)  [unwired: 5 in, 2 out]
    n183 = call-poly <vilib>:"nism.incremental.2.vi"("a phase"=w313, "reset"=w294, "b phase"=w312, "z phase"=w311, "calls per sample"=w341, "index criteria"=w342, "active states"=w343) -> ("encoder position"=w338:i32, "velocity"=w331:i16)  [unwired: 5 in, 2 out]
    n184 = call-poly <vilib>:"nism.incremental.2.vi"("a phase"=w310, "reset"=w294, "b phase"=w309, "z phase"=w308, "calls per sample"=w341, "index criteria"=w342, "active states"=w343) -> ("encoder position"=w337:i32, "velocity"=w330:i16)  [unwired: 5 in, 2 out]
    n185 = call-poly <vilib>:"nism.incremental.2.vi"("a phase"=w297, "reset"=w294, "b phase"=w296, "z phase"=w295, "calls per sample"=w341, "index criteria"=w342, "active states"=w343) -> ("encoder position"=w336:i32, "velocity"=w329:i16)  [unwired: 5 in, 2 out]
    n186 = Build Array(w340, w339, w338, w337, w336) -> (w335:i32[])
    n187 = Build Array(w333, w332, w331, w330, w329) -> (w334:i16[])
    n188 = global write "Global FPGA.vi" "Unfiltered Position Feedback"(w335) -> ()
    n189 = global write "Global FPGA.vi" "Unfiltered Velocity Feedback"(w334) -> ()
  }
  n190 = timed-loop "Synchronization Loop" {
    timing: w7 -> [_]
    timing-out: [_] -> w6
    stop <- FALSE stop-if-true
    n191 = xnode "FPGA I/O Node"() -> ("Scan Clock"=w359:bool)  [unwired: 1 in, 1 out]
    n192 = global read "Global FPGA.vi" "Sync Enable"() -> (w358:bool)
    n193 = Select(t="Sync Value", s="Sync Enable override?", f=w358) -> (s? t:f=w355:bool)
    n194 = call-poly <vilib>:"nism.scan.generateSyncScan.vi"("scan enable?"=w355, "scan clock"=w359) -> ("timer control"=w360:T9)  [unwired: 3 in]
    n195 = global write "Global FPGA.vi" "Timer Control"(w360) -> ()
  }
  n196 = timed-loop "Reset Monitoring Loop" {
    timing: w5 -> [_]
    timing-out: [_] -> w4
    stop <- FALSE stop-if-true
    n197 = global read "Global FPGA.vi" "Reset Pending"() -> (w366:bool[])
    n198 = xnode "FPGA I/O Node"() -> ("Scan Clock"=w365:bool)  [unwired: 1 in, 1 out]
    n199 = feedback-in #1(w365) -> ()
    n200 = feedback #1() -> (w364:bool)  [unwired: 1 in]
    n201 = Greater?(x=w365, y=w364) -> (0:w370:bool)
    n202 = feedback #2() -> (w369:bool[])  [unwired: 1 in]
    n203 = Select(t=w366, s=w370, f=w369) -> (s? t:f=w367:bool[])
    n204 = feedback-in #2(w367) -> ()
    n205 = global write "Global FPGA.vi" "Reset"(w367) -> ()
  }
  n206 = node-c288(w4) -> ()
  n207 = node-c288(w6) -> ()
  n208 = node-c288(w1) -> ()
